vi "Evaluate Part 2.vi"() -> ()   [LabVIEW 2020]
uses:
  Map/Map.lvclass
panel:
  out "Current lowest":u32
  out "Inner":i32
  out "Middle":u32
  out "Outer":i32
  out "lowest":u32
  in  "Input":string="seeds: 79 14 55 13\n\nseed-to-soil map:\n50 98 2\n52 50 48\n\nsoil-to-fertilizer map:\n0 15 37\n37 52 2\n39 0 15\n\nfertilizer-to-water map:\n49 53 8\n0 11 42\n42 0 7\n57 7 4\n\nwater-to-light map:\n88 18 7\n18 25 70\n\nlight-to-temperature map:\n45 77 23\n81 45 19\n68 64 13\n\ntemperature-to-humidity map:\n0 69 1\n1 0 69\n\nhumidity-to-location map:\n60 56 37\n56 93 4"
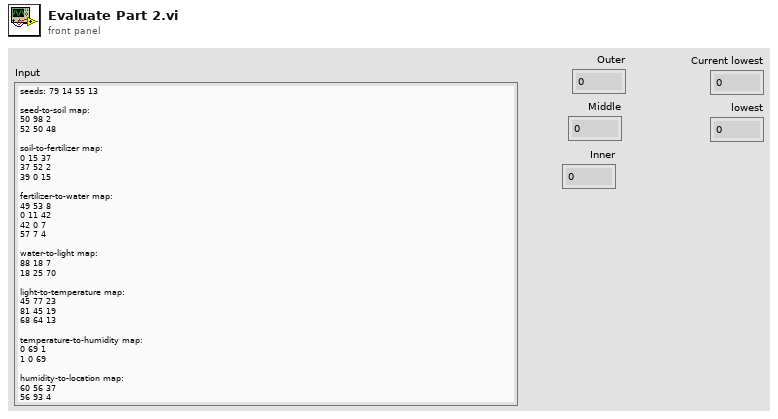
[diagram p1: front panel]
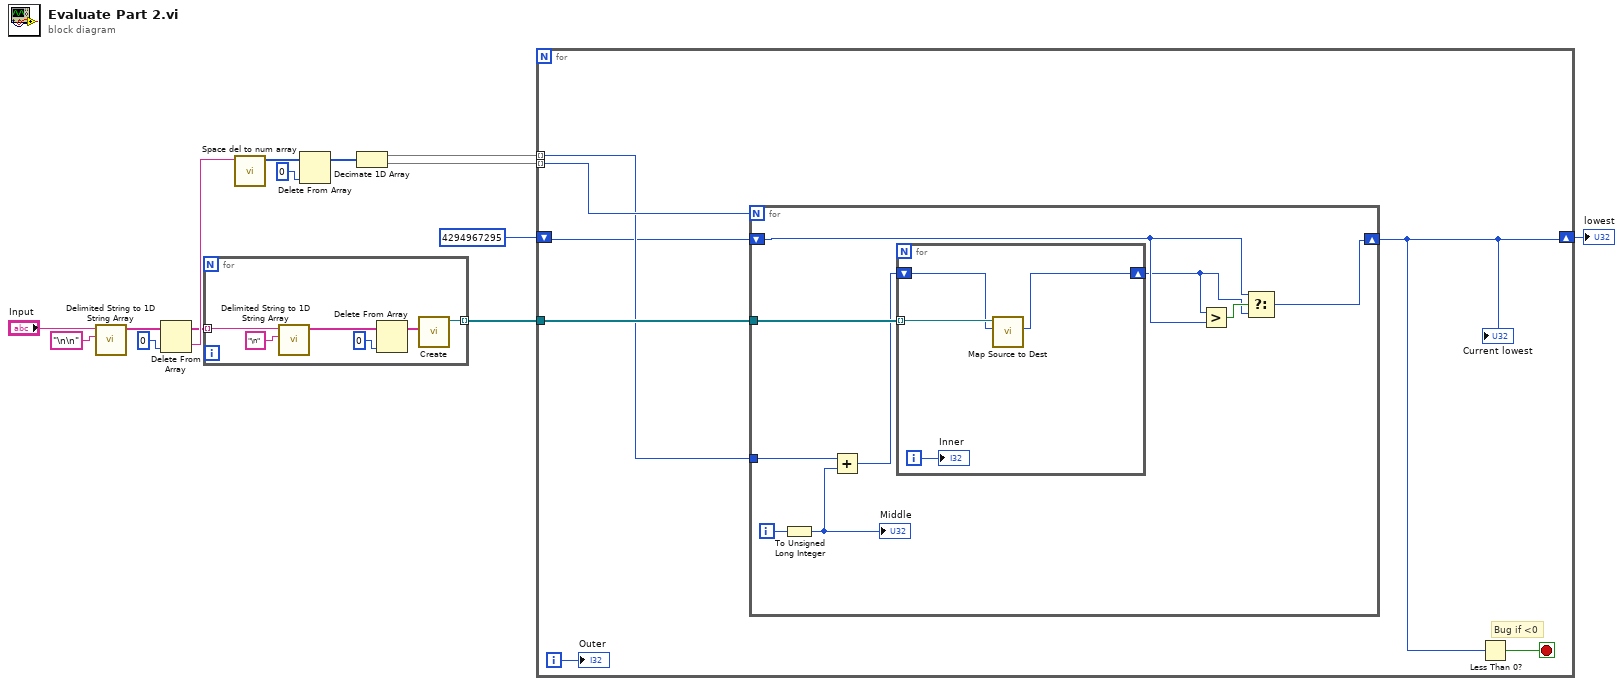
[diagram p0: block diagram]
diagram:
  n1 = call <vilib>:"Delimited String to 1D String Array.vi"("delimiter"="\n\n" ("String"), "delimited string"="Input") -> ("string array"=w8:string[])  [unwired: 9 in]
  n2 = Delete From Array(array=w8, index=0) -> (deleted portion=w11:string, array with subset deleted=w7:string[])  [unwired: 1 in]
  n3 = for {
    tunnel: w7 -> [w18] mode=indexing
    tunnel: [w15] -> w6 mode=indexing
    n4 = call <vilib>:"Delimited String to 1D String Array.vi"("delimiter"="\n" ("String"), "delimited string"=w18) -> ("string array"=w17:string[])  [unwired: 9 in]
    n5 = Delete From Array(array=w17, index=0) -> (array with subset deleted=w16:string[])  [unwired: 1 in, 1 out]
    n6 = call "Create.vi"("Input"=w16) -> ("Map"=w15:refnum<class "Map.lvclass">)  [unwired: 9 in, 1 out]
  }
  n7 = call "Space del to num array.vi"("Input in"=w11) -> ("Input out"=w10:u32[])  [unwired: 10 in]
  n8 = Delete From Array(array=w10, index=0) -> (array with subset deleted=w5:u32[])  [unwired: 1 in, 1 out]
  n9 = Decimate 1D Array(w5) -> (w3:u32[], w4:u32[])
  n10 = for {
    tunnel: w6 -> [w27]
    tunnel: w4 -> [w26] mode=indexing
    tunnel: w3 -> [w25] mode=indexing
    shift-right: [w23] -> w1
    shift-left: u32 4294967295 ("Input") -> [w24]
    i -> [w21]
    stop <- w22 stop-if-true
    # "Bug if <0"
    n11 = for {
      N: w26 -> [_]
      tunnel: w27 -> [w36]
      tunnel: w25 -> [w33]
      shift-right: [w28] -> w23
      shift-left: w24 -> [w30]
      i -> [w34]
      n12 = To Unsigned Long Integer(number=w34) -> (unsigned 32bit integer=w35:u32)
      "Middle" <- w35
      n13 = Add(x=w33, y=w35) -> (x+y=w32:u32)
      n14 = for {
        tunnel: w36 -> [w40] mode=indexing
        shift-right: [w38] -> w29
        shift-left: w32 -> [w39]
        i -> [w37]
        n15 = call "Map Source to Dest.vi"("Source"=w39, "Map in"=w40) -> ("Destination"=w38:u32)  [unwired: 7 in, 2 out]
        "Inner" <- w37
      }
      n16 = Greater?(x=w29, y=w30) -> (0:w31:bool)
      n17 = Select(t=w30, s=w31, f=w29) -> (s? t:f=w28:u32)
    }
    "Current lowest" <- w23
    n18 = Less Than 0?(x=w23) -> (x < 0?=w22:bool)
    "Outer" <- w21
  }
  "lowest" <- w1
